vi "Receive Message.vi"(4 "Paras In":variant, 6 "Priority":i32, 8 "error in (no error)":errorcluster, 9 "Mail Strategy In":refnum<class "Mail Strategy.lvclass">, 10 "Wait(ms)":i32=-1, 11 "Simple Map Queue Group Messenger Component in":refnum<class "Simple Map Queue Group Messenger.lvclass">) -> (0 "error out":errorcluster, 1 "Valid":bool, 2 "Message Out":refnum<class "Message.lvclass">, 3 "Simple Map Queue Group Messenger Component out":refnum<class "Simple Map Queue Group Messenger.lvclass">)   [LabVIEW 2024, in "Simple Map Queue Group Messenger.lvclass"]
uses:
  Simple Map Queue Group Messenger.lvclass
  Ancestor Class/Message/Message.lvclass
  Ancestor Class/Messenger/Mail Strategy/Mail Strategy.lvclass
  Mailman/Simple ID Mailman/Simple ID Mailman.lvclass
  Simple Map Queue Group Messenger.lvclass/Simple Map Queue Group Messenger.ctl
  Mailman/Simple ID Mailman/Simple ID Mailman.lvclass/Simple ID Mailman.ctl
  Mailman/Simple ID Mailman/Public Data/Read ID.vi
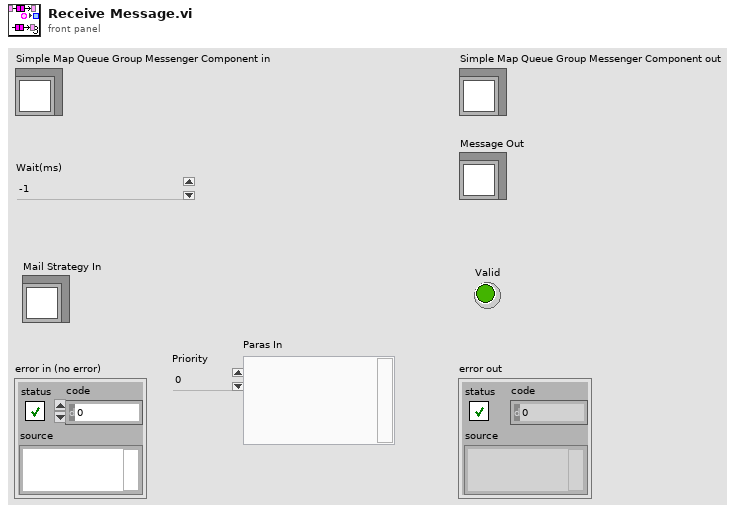
[diagram p1: front panel]
types:
  T1 = typedef "Queue Group Map.ctl" = map{i64, T2[]}
  T2 = typedef "Message Queue.ctl" = refnum<queue>
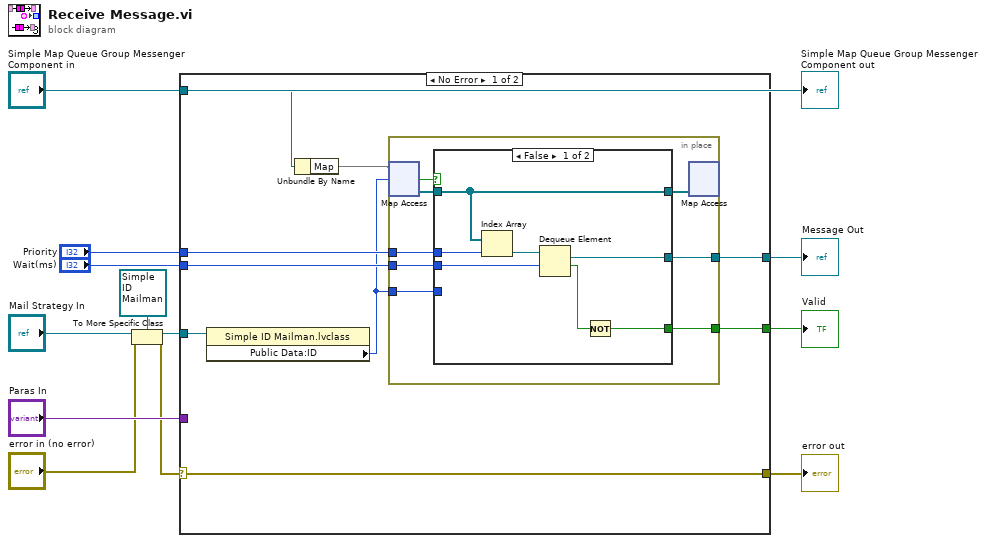
[diagram p0: block diagram]
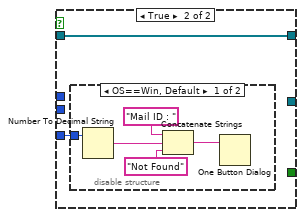
[diagram p2: hidden frame]
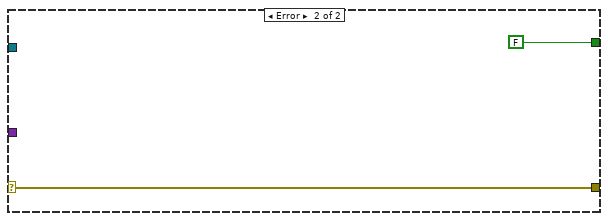
[diagram p4: hidden frame]
diagram:
  n1 = To More Specific Class(target class=refnum<class "Simple ID Mailman.lvclass"> refnum ("Simple ID Mailman.lvclass"), reference="Mail Strategy In", error in="error in (no error)") -> (specific class reference=w3:refnum<class "Simple ID Mailman.lvclass">, error out=w4:errorcluster)
  n2 = case shown="No Error" w4 {
    selector: w4 -> [w14 w45]
    tunnel: "Simple Map Queue Group Messenger Component in" -> [w20 _]
    tunnel: "Paras In" -> [_ _]
    tunnel: "Priority" -> [w19 _]
    tunnel: "Wait(ms)" -> [w18 _]
    tunnel: [w17 _] -> w8
    tunnel: [w16 FALSE] -> w7
    tunnel: w3 -> [w15 _]
    tunnel: [w14 w45] -> w2
    frame No Error {
      n3 = property class="Simple ID Mailman.lvclass"(reference=w15) -> ("Public Data:ID"=w13:i64)  [unwired: 1 in, 2 out]
      n4 = Unbundle By Name(w20) -> ("Map"=w21:T1)
      n5 = in-place {
        in-place-border: w19 -> [w26]
        in-place-border: w18 -> [w25]
        in-place-border: [w24] -> w17
        in-place-border: [w23] -> w16
        in-place-border: w13 -> [w22]
        n6 = in-place-map #1(w21, w13) -> (w28:T2[], w29:bool)  [unwired: 1 in]
        n7 = case shown="False" w29 {
          tunnel: w28 -> [w36 w38]
          tunnel: [w36 w38] -> w27
          tunnel: w26 -> [w34 _]
          tunnel: w25 -> [w33 _]
          tunnel: [w32 _] -> w24
          tunnel: [w30 _] -> w23
          tunnel: w22 -> [_ w37]
          frame False {
            n8 = Index Array(array=w36, index=w34) -> (element=w35:T2)
            n9 = Dequeue Element(queue=w35, timeout in ms (-1)=w33) -> (element=w32:refnum<class "Message.lvclass">, timed out?=w31:bool)  [unwired: 1 in, 2 out]
            n10 = Not(x=w31) -> (.not. x?=w30:bool)
          }
          frame True {
            n11 = disable-structure shown="OS==Win, Default" {
              disable-tunnel: w37 -> [w43 _]
              frame condition #0 (active) {
                n12 = Number To Decimal String(number=w43) -> (decimal integer string=w41:string)  [unwired: 1 in]
                n13 = Concatenate Strings("Mail ID : " ("message"), w41, "Not Found" ("message")) -> (w39:string)
                n14 = One Button Dialog(message=w39) -> ()  [unwired: 1 in, 1 out]
              }
              frame condition #1 {
              }
            }
          }
        }
        n15 = in-place-map #1(w27) -> ()  [unwired: 1 in, 3 out]
      }
    }
    frame Error {
    }
  }
  "error out" <- w2
  "Message Out" <- w8
  "Valid" <- w7
  "Simple Map Queue Group Messenger Component out" <- "Simple Map Queue Group Messenger Component in"
